vi "Shutdown.vi"(8 "error in (no error)":errorcluster, 11 "Thread in":refnum<class "Thread.lvclass">) -> (0 "error out":errorcluster, 3 "Thread out":refnum<class "Thread.lvclass">)   [LabVIEW 2017, in "DSF Core.lvlib" / "Thread.lvclass"]
uses:
  Thread.lvclass
  Thread Command.ctl
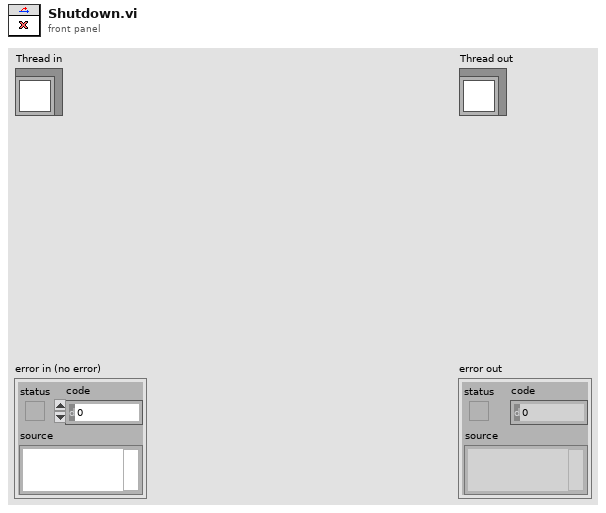
[diagram p1: front panel]
types:
  T1 = typedef "DSF Core.lvlib/Thread.lvclass/Thread State.ctl" = enum8{"Idle", "Running", "Error", "Shut Down"}
  T2 = typedef "DSF Core.lvlib/Thread.lvclass/Thread Command.ctl" = enum8{"Run", "Shutdown"}
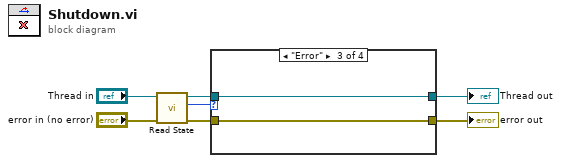
[diagram p0: block diagram]
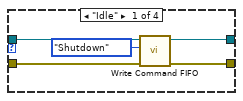
[diagram p2: hidden frame]
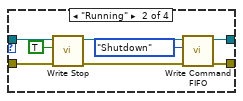
[diagram p3: hidden frame]
diagram:
  n1 = call "Read State.vi"("error in (no error)"="error in (no error)", "Thread in"="Thread in") -> ("error out"=w6:errorcluster, "state"=w5:T1, "Thread out"=w7:refnum<class "Thread.lvclass">)  [unwired: 7 in]
  n2 = case shown="\"Error\"" w5 {
    tunnel: w7 -> [w12 w20 w22 w23]
    tunnel: w6 -> [w11 w19 w21 w24]
    tunnel: [w10 w14 w22 w23] -> w2
    tunnel: [w9 w15 w21 w24] -> w1
    frame "Idle" {
      n3 = call "Write Command FIFO.vi"("error in (no error)"=w11, "command"=Thread_Command."Shutdown", "Thread in"=w12) -> ("error out"=w9:errorcluster, "Thread out"=w10:refnum<class "Thread.lvclass">)  [unwired: 5 in, 2 out]
    }
    frame "Running" {
      n4 = call "Write Stop.vi"("error in (no error)"=w19, "stop"=TRUE, "Thread in"=w20) -> ("error out"=w16:errorcluster, "Thread out"=w13:refnum<class "Thread.lvclass">)  [unwired: 7 in]
      n5 = call "Write Command FIFO.vi"("error in (no error)"=w16, "command"=Thread_Command."Shutdown", "Thread in"=w13) -> ("error out"=w15:errorcluster, "Thread out"=w14:refnum<class "Thread.lvclass">)  [unwired: 5 in, 2 out]
    }
    frame "Error" {
    }
    frame "Shut Down" {
    }
  }
  "error out" <- w1
  "Thread out" <- w2
